vi "gotoTopBotExp.vi"(8 "error in (no error)":errorcluster, 9 "position":refnum<vi>, 10 "motor setting":refnum<vi>, 11 "appended array":refnum<k7>[](array[refnum])) -> (0 "error out":errorcluster)   [LabVIEW 2014]
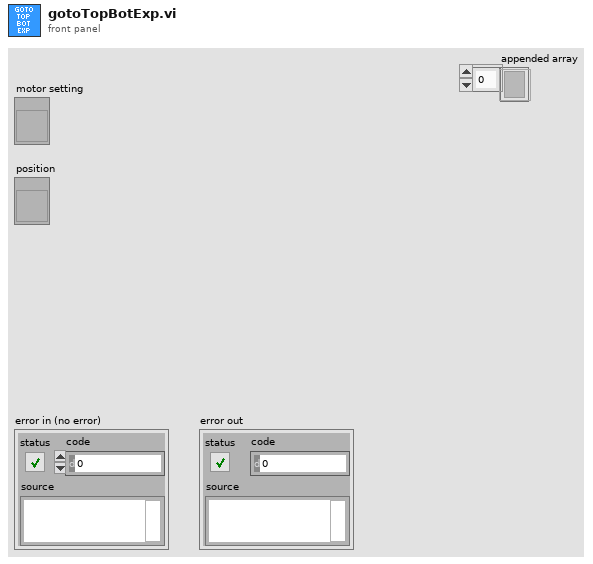
[diagram p1: front panel]
types:
  T1 = cluster{"X Acc (mm/s^2)":sgl, "X Vmax (mm/s)":sgl, "Y Acc (mm/s^2)":sgl, "Y Vmax (mm/s)":sgl, "Z Acc (mm/s^2)":sgl, "Z Vmax (mm/s)":sgl}
  T2 = cluster{"X Pos (mm)":sgl, "Y Pos (mm)":sgl, "Z Pos (mm)":sgl}
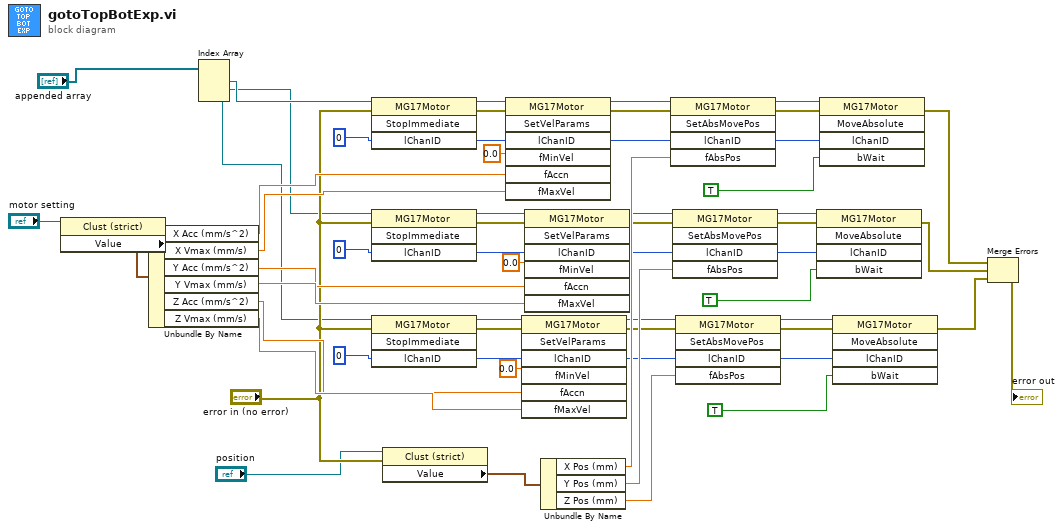
[diagram p0: block diagram]
diagram:
  n1 = property on="Property Node" class="Clust (strict)"(reference="motor setting") -> ("Value"=w24:T1)  [unwired: 1 in, 2 out]
  n2 = Unbundle By Name(w24) -> ("X Acc (mm/s^2)"=w25:sgl, "X Vmax (mm/s)"=w26:sgl, "Y Acc (mm/s^2)"=w27:sgl, "Y Vmax (mm/s)"=w28:sgl, "Z Acc (mm/s^2)"=w29:sgl, "Z Vmax (mm/s)"=w30:sgl)
  n3 = Index Array(array="appended array") -> (element #1=w18:refnum<k7>, element #2=w17:refnum<k7>, element #3=w16:refnum<k7>)  [unwired: 3 in]
  n4 = invoke class="MG17Motor" method="StopImmediate"(reference=w18, error in="error in (no error)", "lChanID"=0) -> (reference out=w34:refnum<k7>, error out=w33:errorcluster, "lChanID"=w54:i32)  [unwired: 1 in, 1 out]
  n5 = invoke class="MG17Motor" method="StopImmediate"(reference=w17, error in="error in (no error)", "lChanID"=0) -> (reference out=w40:refnum<k7>, error out=w39:errorcluster, "lChanID"=w53:i32)  [unwired: 1 in, 1 out]
  n6 = invoke class="MG17Motor" method="StopImmediate"(reference=w16, error in="error in (no error)", "lChanID"=0) -> (reference out=w47:refnum<k7>, error out=w46:errorcluster, "lChanID"=w52:i32)  [unwired: 1 in, 1 out]
  n7 = property on="Property Node" class="Clust (strict)"(reference="position", error in="error in (no error)") -> ("Value"=w31:T2)  [unwired: 2 out]
  n8 = invoke class="MG17Motor" method="SetVelParams"(reference=w34, error in=w33, "lChanID"=w54, "fMinVel"=sgl 0.0, "fAccn"=w25, "fMaxVel"=w26) -> (reference out=w35:refnum<k7>, error out=w36:errorcluster, "lChanID"=w37:i32)  [unwired: 1 in, 4 out]
  n9 = invoke class="MG17Motor" method="SetVelParams"(reference=w47, error in=w46, "lChanID"=w52, "fMinVel"=sgl 0.0, "fAccn"=w29, "fMaxVel"=w30) -> (reference out=w48:refnum<k7>, error out=w49:errorcluster, "lChanID"=w50:i32)  [unwired: 1 in, 4 out]
  n10 = invoke class="MG17Motor" method="SetVelParams"(reference=w40, error in=w39, "lChanID"=w53, "fMinVel"=sgl 0.0, "fAccn"=w27, "fMaxVel"=w28) -> (reference out=w42:refnum<k7>, error out=w43:errorcluster, "lChanID"=w44:i32)  [unwired: 1 in, 4 out]
  n11 = Unbundle By Name(w31) -> ("X Pos (mm)"=w56:sgl, "Y Pos (mm)"=w57:sgl, "Z Pos (mm)"=w58:sgl)
  n12 = invoke class="MG17Motor" method="SetAbsMovePos"(reference=w35, error in=w36, "lChanID"=w37, "fAbsPos"=w56) -> (reference out=w15:refnum<k7>, error out=w14:errorcluster, "lChanID"=w11:i32)  [unwired: 1 in, 2 out]
  n13 = invoke class="MG17Motor" method="SetAbsMovePos"(reference=w42, error in=w43, "lChanID"=w44, "fAbsPos"=w57) -> (reference out=w10:refnum<k7>, error out=w9:errorcluster, "lChanID"=w7:i32)  [unwired: 1 in, 2 out]
  n14 = invoke class="MG17Motor" method="SetAbsMovePos"(reference=w48, error in=w49, "lChanID"=w50, "fAbsPos"=w58) -> (reference out=w4:refnum<k7>, error out=w5:errorcluster, "lChanID"=w2:i32)  [unwired: 1 in, 2 out]
  n15 = invoke class="MG17Motor" method="MoveAbsolute"(reference=w10, error in=w9, "lChanID"=w7, "bWait"=TRUE) -> (error out=w8:errorcluster)  [unwired: 1 in, 4 out]
  n16 = invoke class="MG17Motor" method="MoveAbsolute"(reference=w15, error in=w14, "lChanID"=w11, "bWait"=TRUE) -> (error out=w13:errorcluster)  [unwired: 1 in, 4 out]
  n17 = invoke class="MG17Motor" method="MoveAbsolute"(reference=w4, error in=w5, "lChanID"=w2, "bWait"=TRUE) -> (error out=w3:errorcluster)  [unwired: 1 in, 4 out]
  n18 = Merge Errors(w13, w8, w3) -> (→"error out":errorcluster)
